vi "GageAverage.vi"() -> ()   [LabVIEW 2016]
uses:
  <vilib>/express/express analysis/Spectral/Block/exnSpectralBlock spectral measurements power poly.vi
  <vilib>/express/express analysis/Spectral/Block/exnSpectralBlock spectral measurements power WFM.vi
  <vilib>/Utility/file.llb/Write To Spreadsheet File (DBL).vi
  <vilib>/Analysis/2dsp.llb/1D Cross Correlation (DBL).vi
  <vilib>/express/express analysis/Spectral/XNode/ExpressSpectralMeasurementsBlockNode.xnode
  <vilib>/Analysis/NI_AALPro.lvlib
panel:
  out "100 세트 저장완료":bool
  in  "데이터 저장 시작":bool
  out "루프 사이의 time interval":dbl
  out "Ant 3":dbl(graph)
  out "ANt 2":dbl(graph)
  out "Ant 1":dbl(graph)
  in  "상호상관 샘플 갯수":dbl
  in  "상호상관\n채널 2":i32=1
  in  "상호상관 채널 1":i32=1
  out "웨이브폼 그래프 2":dbl[](graph)
  in  "표시 채널":i32=1
  out "웨이브폼 그래프":cluster{"f0":dbl, "df":dbl, "magnitude":dbl[]}(graph)
  in  "Trigger":T1={"Slope"=0, "Level"=0, "Source"=0, "External Range"=2000, "External Coupling"=0, "External"=FALSE, "Disable"=FALSE, "External Impedance"=1} {"External Impedance" items=["50 Ohm", "HiZ"]; "External Coupling" items=["DC", "AC"]; "External Range" min=2000 max=10000 step=8000; "Slope" items=["Rising", "Falling"]; "Level" min=-100 max=100; "Source" min=0 max=64 step=1}
  in  "Averages":u32=1 min=1 step=1
  in  "Averaging Method":bool
  in  "Channels":T2(array[cluster])=[{"Coupling"=0, "Differential Input"=FALSE, "Direct-to-ADC"=FALSE, "Range"=2000, "Impedance"=50, "Filter"=0}] {"Impedance" min=50 max=1000000 step=999950; "Coupling" items=["DC", "AC"]}
  in  "Acquisition":T3={"Sample Rate"=50000000.0, "Mode"=2, "Depth"=8192.0, "Segment Size"=8192.0, "Trigger Timeout"=1000000.0, "Trigger Holdoff"=0.0, "Trigger Delay"=0.0, "Clock mode"=enum."Internal"} {"Segment Size" min=256.0 step=128.0; "Trigger Holdoff" min=0.0 step=128.0; "Trigger Delay" min=0.0 step=128.0; "Depth" min=256.0 step=128.0; "Mode" items=["Single", "Dual", "Quad", "Octal"]}
  in  "Continuous":bool=TRUE
  out "Progress":string
  in  "stop":bool
  out "Waveform Graph":cluster{dbl, dbl, dbl[]}(graph)
  out "System Name":string
  out "Sample Bits":i32
  out "Trigger Count":i32
  out "Channel Count":i32
  out "Board Count":i32
  out "System Count":i32
  in  "Points":u32=4096
  in  "Start":i32
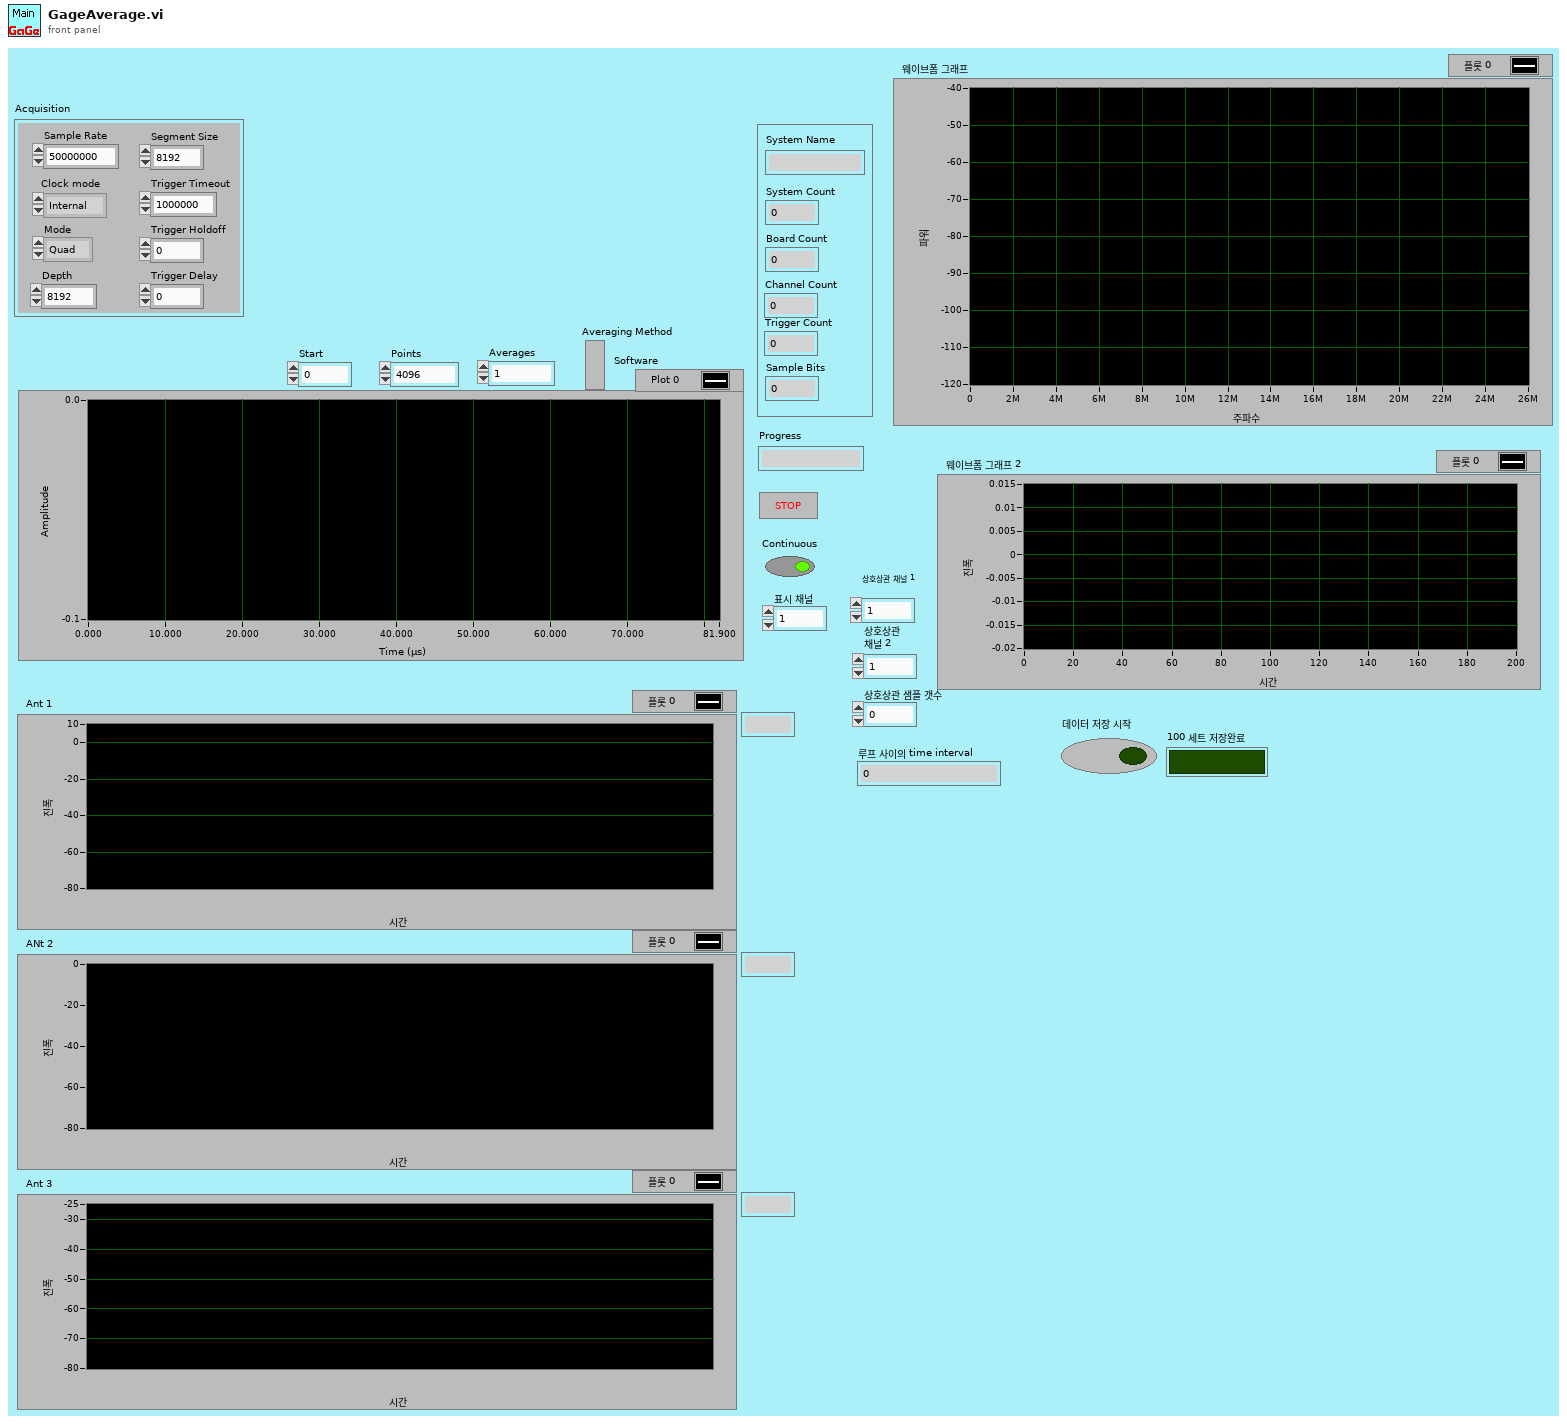
[diagram p1: front panel]
types:
  T1 = cluster{"Slope":u16, "Level":i32, "Source":i32, "External Range":u32, "External Coupling":u16, "External":bool, "Disable":bool, "External Impedance":u16}
  T2 = cluster{"Coupling":u16, "Differential Input":bool, "Direct-to-ADC":bool, "Range":u32, "Impedance":u32, "Filter":i32}[]
  T3 = cluster{"Sample Rate":dbl, "Mode":u16, "Depth":dbl, "Segment Size":dbl, "Trigger Timeout":dbl, "Trigger Holdoff":dbl, "Trigger Delay":dbl, "Clock mode":enum16{"Internal", "External", "Reference"}}
  T4 = cluster{"averaging mode":u16, "weighting mode":u16, "number of averages":u32}
  T5 = cluster{"dB On (F)":bool, "unwrap phase (F)":bool, "convert to degree (F)":bool}
  T6 = cluster{"Handle":u32, "Sample size":u32, "Resolution":i32, "Offset":i32, "Channels":u32, "Boards":u32}
  T7 = cluster{string, "Differential Input":bool, "Direct-to-ADC":bool, "Range":u32, "Impedance":u32, i32, "Filter":i32}
  T8 = cluster{"RingText.Text":string, "Level":i32, "Source":i32, "External Range":u32, "RingText.Text":string, "External":bool, "Disable":bool, "RingText.Text":string}
  T9 = cluster{"RingText.Text":string, "Level":i32, "Source":i32, "External Range":u32, "RingText.Text":string, "External":bool, "Disable":bool, "RingText.Text":string}[]
  T10 = cluster{"Handle":u32, "Sample Size":u32, "Resolution":i32, "Offset":i32, "Channels":u32, "Boards":u32}
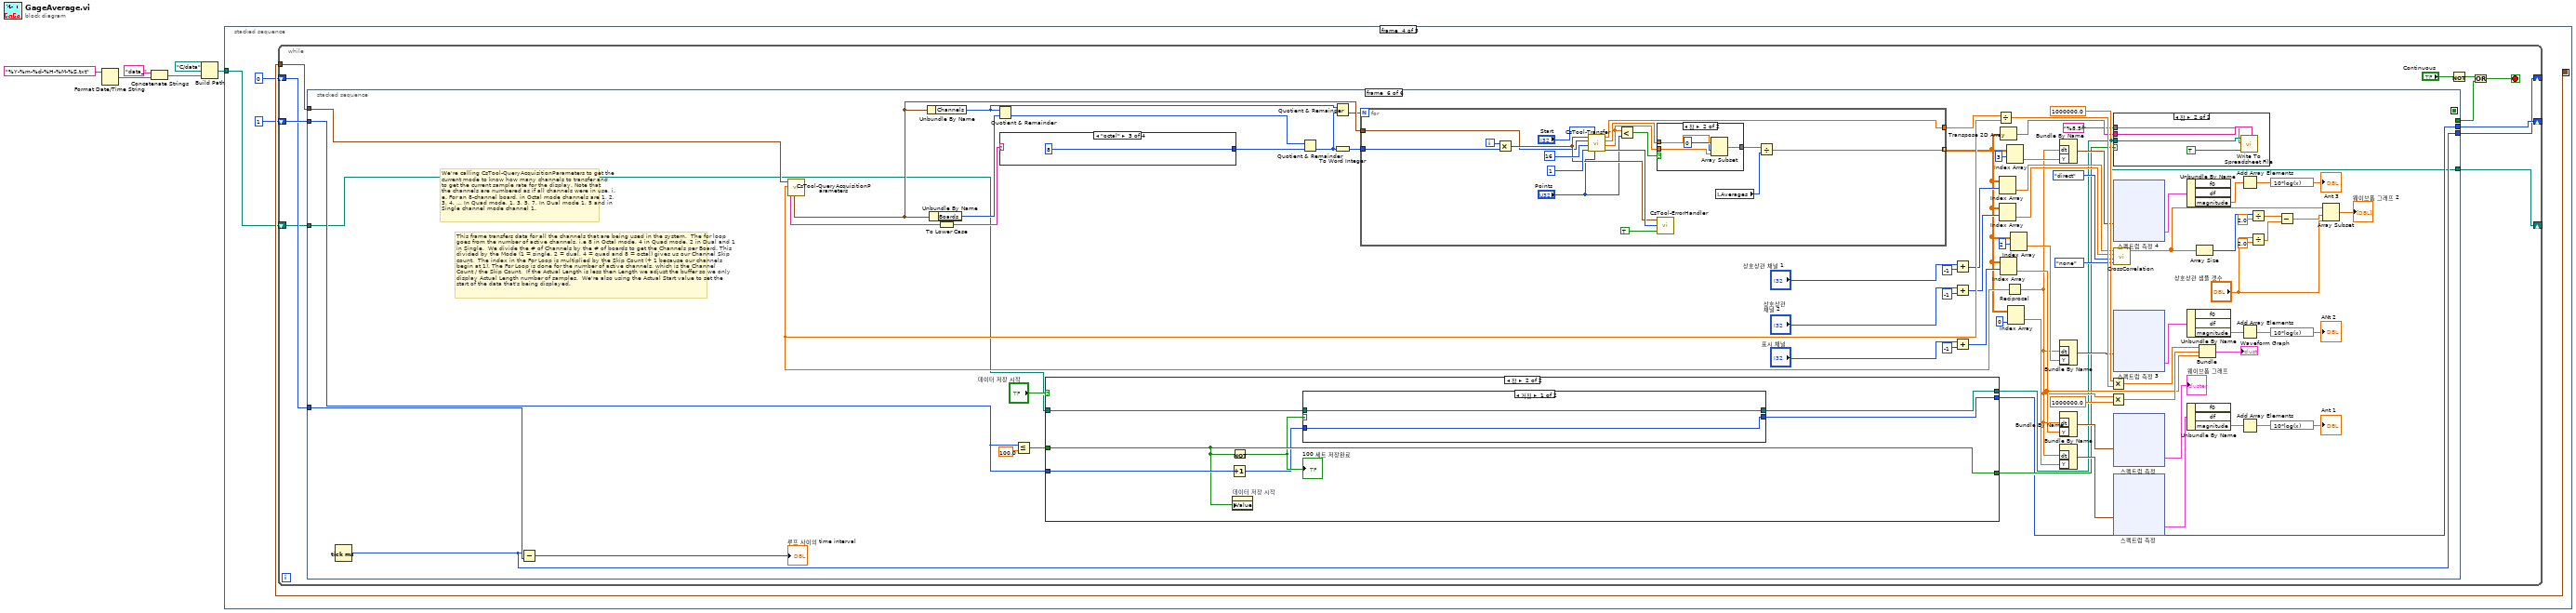
[diagram p0: block diagram]
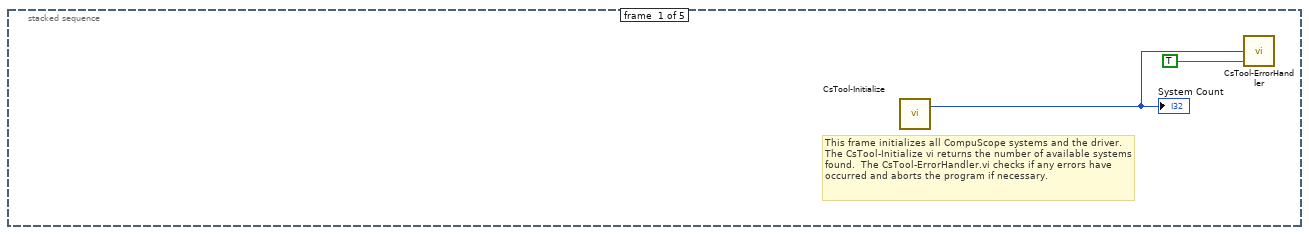
[diagram p2: hidden frame]
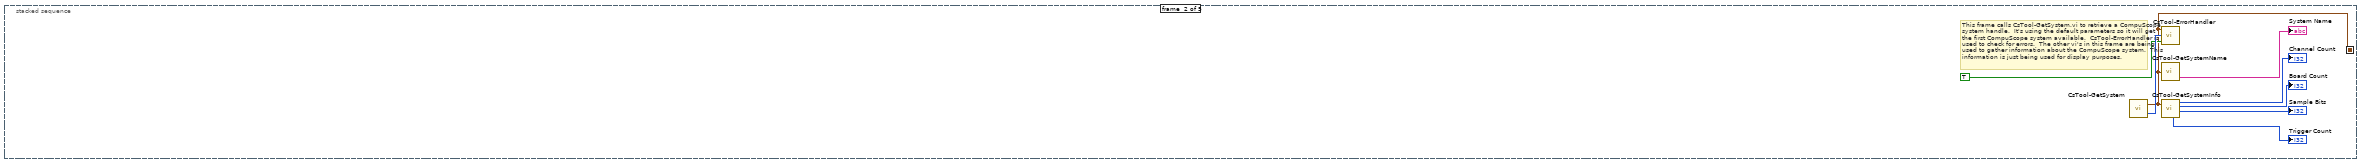
[diagram p3: hidden frame]
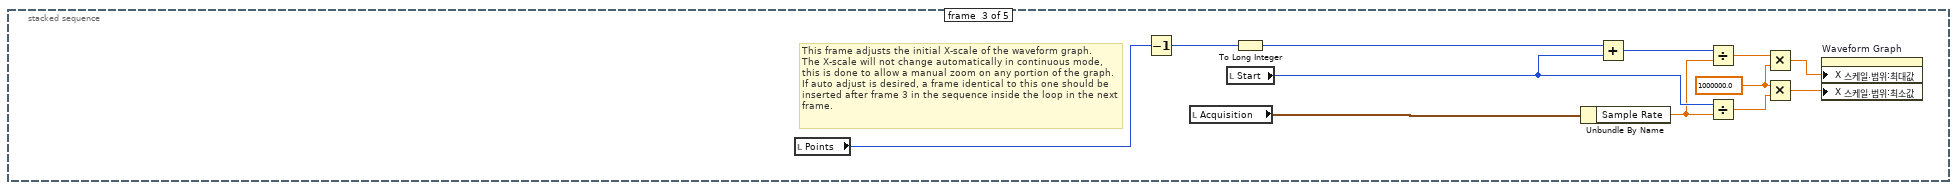
[diagram p4: hidden frame]
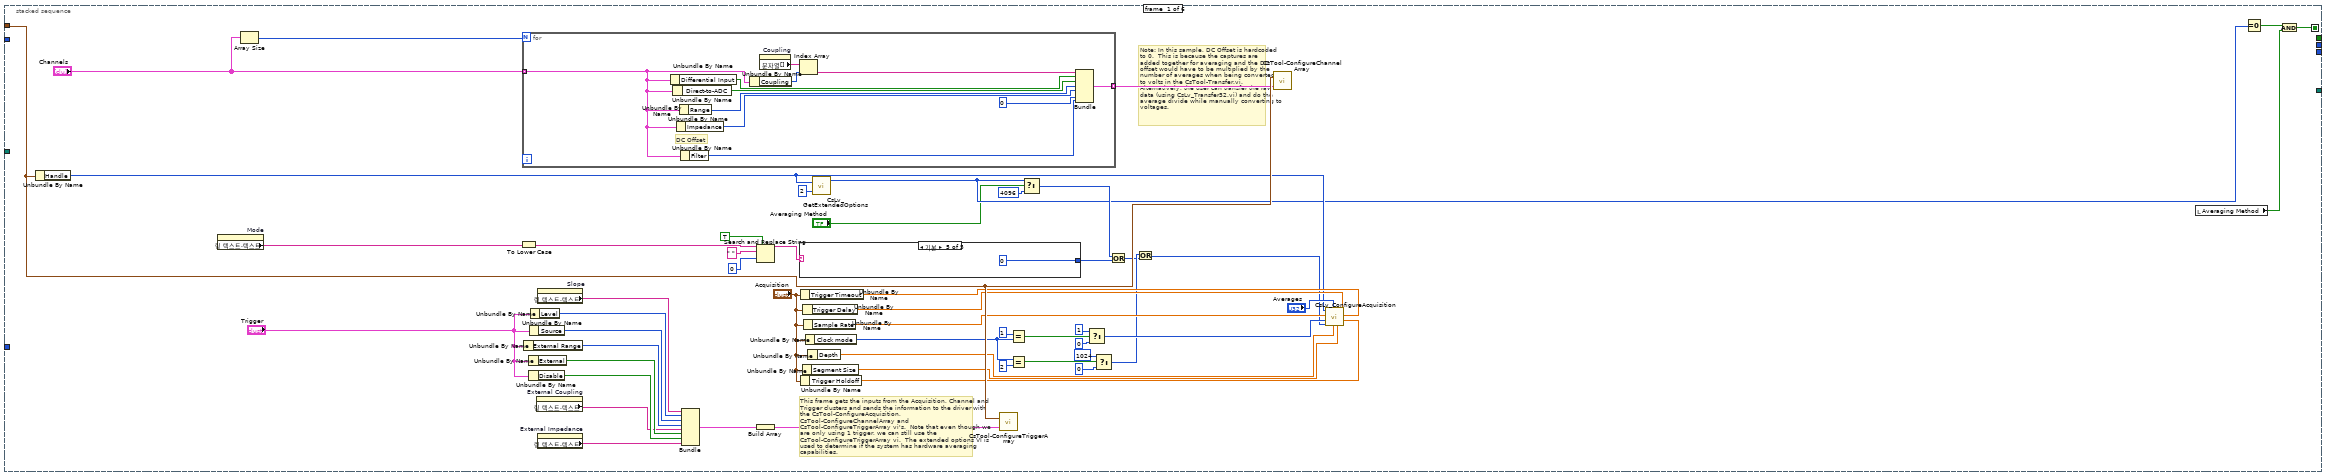
[diagram p5: hidden frame]
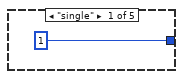
[diagram p6: hidden frame]
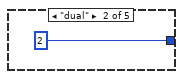
[diagram p7: hidden frame]
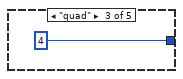
[diagram p8: hidden frame]
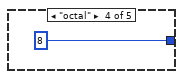
[diagram p9: hidden frame]
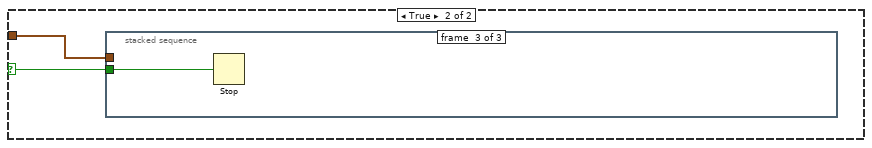
[diagram p11: hidden frame]
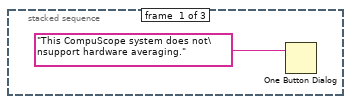
[diagram p12: hidden frame]
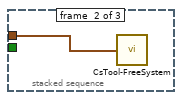
[diagram p13: hidden frame]
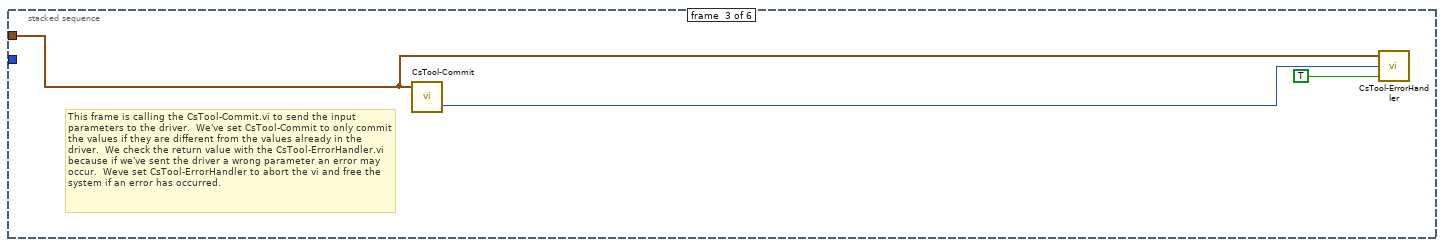
[diagram p14: hidden frame]
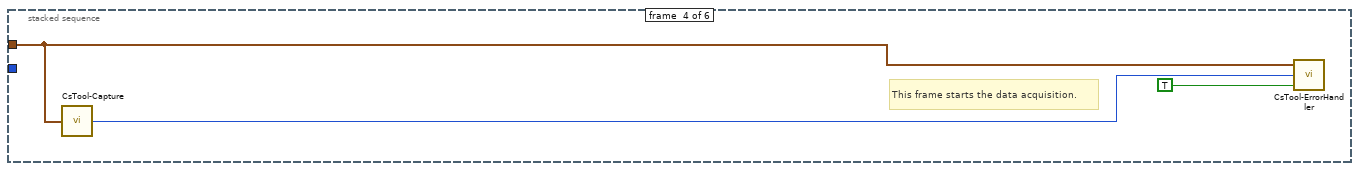
[diagram p15: hidden frame]
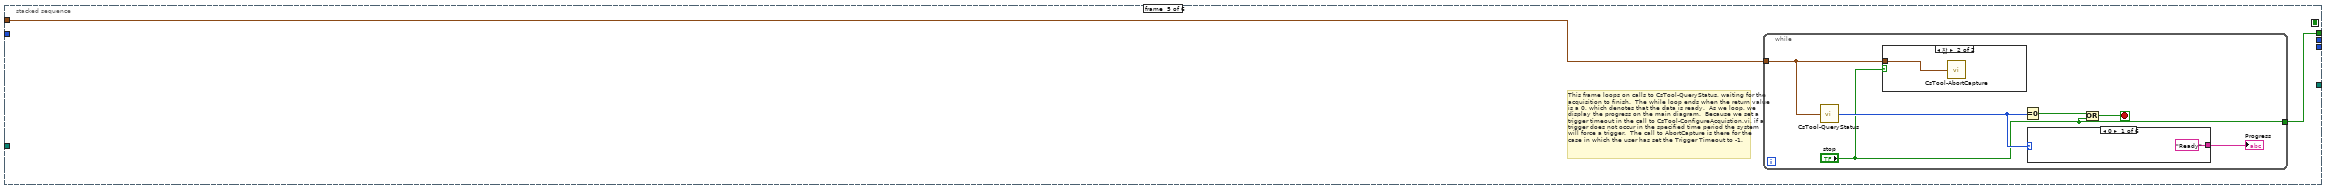
[diagram p16: hidden frame]
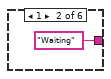
[diagram p18: hidden frame]
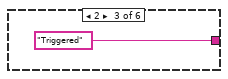
[diagram p19: hidden frame]
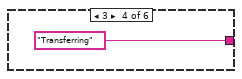
[diagram p20: hidden frame]
diagram:
  n1 = Format Date/Time String(time format string (%c)="%Y-%m-%d-%H-%M-%S.txt" ("시간 포맷 문자열 (%c)")) -> (date/time string=w2:string)  [unwired: 2 in]
  n2 = Concatenate Strings("data_", w2) -> (w1:string)
  n3 = Build Path(base path=path "C:/data", name or relative path=w1) -> (appended path=w4:path)
  n4 = stacked-sequence {
    seq-local: [_ w11 _ _ _] -> [_ _ _ w32 w305]
    tunnel: w4 -> [_ _ _ w29 _]
    frame #0 {
      # "This frame initializes all CompuScope systems and the driver.\nThe CsTool-Initialize vi returns the number of available systems found.  The CsTool-ErrorHandler.vi checks if any errors have occurred and aborts the program if necessary."
      n5 = call <userlib>:"CsTool-Initialize.vi"() -> ("Number Of Systems"=w8:i32)  [unwired: 1 out]
      "System Count" <- w8
      n6 = call <userlib>:"CsTool-ErrorHandler.vi"("StopOnError (true)"=TRUE, "Error Code"=w8) -> ()  [unwired: 1 in, 1 out]
    }
    frame #1 {
      # "This frame calls CsTool-GetSystem.vi to retrieve a CompuScope system handle.  It's using the default parameters so it will get the first CompuScope system available.  CsTool-ErrorHandler is used to check for errors.  The other vi's in this frame are being used to gather information about the CompuScope system.  This information is just being used for display purposes."
      n7 = call <userlib>:"CsTool-GetSystem.vi"() -> ("Error Code"=w13:i32, "Handle Cluster"=w11:T6)  [unwired: 4 in]
      n8 = call <userlib>:"CsTool-ErrorHandler.vi"("StopOnError (true)"=TRUE, "Error Code"=w13, "Handle Cluster"=w11) -> ()  [unwired: 1 out]
      n9 = call <userlib>:"CsTool-GetSystemName.vi"("Handle Cluster"=w11) -> ("System Name"=→"System Name":string)  [unwired: 1 out]
      n10 = call <userlib>:"CsTool-GetSystemInfo.vi"("Handle Cluster"=w11) -> ("Number Of Triggers"=→"Trigger Count":u32, "Number Of Channels"=→"Channel Count":u32, "Number Of Boards"=→"Board Count":u32, "Sample Bits"=→"Sample Bits":u32)  [unwired: 3 out]
    }
    frame #2 {
      w28 = 1000000.0
      # "This frame adjusts the initial X-scale of the waveform graph.\nThe X-scale will not change automatically in continuous mode, \nthis is done to allow a manual zoom on any portion of the graph.\nIf auto adjust is desired, a frame identical to this one should be\ninserted after frame 3 in the sequence inside the loop in the next frame."
      n11 = local read "Points"() -> (w23:u32)
      n12 = Decrement(x=w23) -> (x-1=w17:u32)
      n13 = local read "Acquisition"() -> (w21:T3)
      n14 = local read "Start"() -> (w24:i32)
      n15 = To Long Integer(number=w17) -> (32bit integer=w18:i32)
      n16 = Unbundle By Name(w21) -> ("Sample Rate"=w22:dbl)
      n17 = Add(x=w18, y=w24) -> (x+y=w20:i32)
      n18 = Divide(x=w20, y=w22) -> (x/y=w19:dbl)
      n19 = Divide(x=w24, y=w22) -> (x/y=w27:dbl)
      n20 = Multiply(x=w19, y=w28) -> (x*y=w25:dbl)
      n21 = Multiply(x=w28, y=w27) -> (x*y=w26:dbl)
      n22 = property on="Waveform Graph" class="WFGraph (엄격한)"("X 스케일.범위:최대값"=w25, "X 스케일.범위:최소값"=w26) -> ()  [unwired: 2 in, 2 out]
    }
    frame #3 {
      n23 = while {
        tunnel: w32 -> [w43]
        shift-right: [w37] -> _
        shift-left: 1 -> [w38]
        shift-right: [w35] -> _
        shift-left: 0 -> [w36]
        shift-right: [w34] -> _
        shift-left: w29 -> [w33]
        stop <- w40 stop-if-true
        n24 = stacked-sequence {
          seq-local: [w64 _ _ _ _ _] -> [_ w113 _ _ _ _]
          tunnel: w43 -> [w89 w112 w119 w122 w126 w219]
          tunnel: [_ _ _ _ w125 _] -> w39
          tunnel: w38 -> [_ _ _ _ _ w149]
          tunnel: [_ _ _ _ _ w150] -> w37
          tunnel: w36 -> [_ _ _ _ _ w156]
          tunnel: [_ _ _ _ _ w154] -> w35
          tunnel: [_ _ _ _ _ w144] -> w34
          tunnel: w33 -> [_ _ _ _ _ w143]
          frame #0 {
            # "Note: In this sample, DC Offset is hardcoded to 0.  This is because the captures are added together for averaging and the DC offset would have to be multiplied by the number of averages when being converted to volts in the CsTool-Transfer.vi. Alternatively, the user can transfer the raw data (using CsLv_Transfer32.vi) and do the average divide while manually converting to voltages."
            # "This frame gets the inputs from the Acquisition, Channel and Trigger clusters and sends the information to the driver with the CsTool-ConfigureAcquisition, CsTool-ConfigureChannelArray and CsTool-ConfigureTriggerArray vi's.  Note that even though we are only using 1 trigger, we can still use the CsTool-ConfigureTriggerArray vi.  The extended options VI is used to determine if the system has hardware averaging capabilities."
            n25 = Unbundle By Name(w89) -> ("Handle"=w68:u32)
            n26 = property on="Mode" class="Ring (엄격한)"() -> ("링 텍스트.텍스트"=w78:string)  [unwired: 2 in, 2 out]
            n27 = Array Size(array="Channels") -> (size(s)=w90:i32)
            n28 = To Lower Case(string=w78) -> (all lower case string=w84:string)
            n29 = for {
              N: w90 -> [_]
              tunnel: "Channels" -> [w103] mode=indexing
              tunnel: [w107] -> w48 mode=indexing
              # "DC Offset"
              n30 = Unbundle By Name(w103) -> ("Differential Input"=w111:bool)
              n31 = Unbundle By Name(w103) -> ("Direct-to-ADC"=w110:bool)
              n32 = Unbundle By Name(w103) -> ("Impedance"=w108:u32)
              n33 = Unbundle By Name(w103) -> ("Range"=w109:u32)
              n34 = Unbundle By Name(w103) -> ("Filter"=w102:i32)
              n35 = Unbundle By Name(w103) -> ("Coupling"=w105:u16)
              n36 = property on="Coupling" class="Ring (엄격한)"() -> ("문자열[]"=w106:string[])  [unwired: 2 in, 2 out]
              n37 = Index Array(array=w106, index=w105) -> (element=w104:string)
              n38 = Bundle(w104, "Differential Input"=w111, "Direct-to-ADC"=w110, "Range"=w109, "Impedance"=w108, 0, "Filter"=w102) -> (w107:T7)  [unwired: 1 in]
            }
            n39 = Unbundle By Name("Trigger") -> ("External Range"=w94:u32)
            n40 = Unbundle By Name("Trigger") -> ("External"=w50:bool)
            n41 = Unbundle By Name("Trigger") -> ("Disable"=w49:bool)
            n42 = Unbundle By Name("Trigger") -> ("Source"=w51:i32)
            n43 = Unbundle By Name("Trigger") -> ("Level"=w95:i32)
            n44 = property on="External Coupling" class="Ring (엄격한)"() -> ("링 텍스트.텍스트"=w45:string)  [unwired: 2 in, 2 out]
            n45 = property on="Slope" class="Ring (엄격한)"() -> ("링 텍스트.텍스트"=w46:string)  [unwired: 2 in, 2 out]
            n46 = property on="External Impedance" class="Ring (엄격한)"() -> ("링 텍스트.텍스트"=w44:string)  [unwired: 2 in, 2 out]
            n47 = Bundle("RingText.Text"=w46, "Level"=w95, "Source"=w51, "External Range"=w94, "RingText.Text"=w45, "External"=w50, "Disable"=w49, "RingText.Text"=w44) -> (w93:T8)  [unwired: 1 in]
            n48 = Search and Replace String(replace all?=TRUE, input string=w84, search string=" ", offset=0) -> (result string=w81:string)  [unwired: 4 in, 3 out]
            n49 = Build Array(w93) -> (w92:T9)
            n50 = case shown="기본" w81 {
              tunnel: [1 2 4 8 0] -> w69
              frame "single" {
              }
              frame "dual" {
              }
              frame "quad" {
              }
              frame "octal" {
              }
              frame Default {
              }
            }
            n51 = Unbundle By Name("Acquisition") -> ("Trigger Timeout"=w75:dbl)
            n52 = Unbundle By Name("Acquisition") -> ("Trigger Holdoff"=w74:dbl)
            n53 = Unbundle By Name("Acquisition") -> ("Segment Size"=w77:dbl)
            n54 = Unbundle By Name("Acquisition") -> ("Trigger Delay"=w76:dbl)
            n55 = Unbundle By Name("Acquisition") -> ("Sample Rate"=w88:dbl)
            n56 = Unbundle By Name("Acquisition") -> ("Clock mode"=w59:enum16{"Internal", "External", "Reference"})
            n57 = Unbundle By Name("Acquisition") -> ("Depth"=w80:dbl)
            n58 = call <userlib>:"CsLv_GetExtendedOptions.vi"("Handle"=w68, "Option"=2) -> ("User Mode"=w66:u32)  [unwired: 2 out]
            n59 = call <userlib>:"CsTool-ConfigureTriggerArray.vi"("Triggers"=w92, "Handle Cluster"=w89) -> ()  [unwired: 1 out]
            n60 = Equal?(x=1, y=w59) -> (x = y?=w60:bool)
            n61 = Equal?(x=w59, y=2) -> (x = y?=w57:bool)
            n62 = Select(t=w66, s="Averaging Method", f=4096) -> (s? t:f=w70:u32)
            n63 = Select(t=u32 1, s=w60, f=u32 0) -> (s? t:f=w85:u32)
            n64 = Select(t=1024, s=w57, f=0) -> (s? t:f=w56:i32)
            n65 = Or(x=w70, y=w69) -> (x .or. y?=w54:u32)
            n66 = Or(x=w56, y=w54) -> (x .or. y?=w55:u32)
            n67 = call <userlib>:"CsTool-ConfigureChannelArray.vi"("Channels"=w48, "Handle Cluster"=w89) -> ()  [unwired: 1 out]
            n68 = call <userlib>:"CsLv_ConfigureAcquisition.vi"("Trigger Holdoff (0)"=w74, "Trigger Timeout (10000000)"=w75, "Trigger Delay (0)"=w76, "Segment Size (8192)"=w77, "Depth (8192)"=w80, "Segment Count (1)"="Averages", "Mode (2)"=w55, "External Clock (0)"=w85, "Sample Rate (100000000)"=w88, "Handle"=w68) -> ()  [unwired: 1 in, 1 out]
            n69 = local read "Averaging Method"() -> (w53:bool)
            n70 = Equal To 0?(x=w66) -> (x = 0?=w65:bool)
            n71 = And(x=w65, y=w53) -> (x .and. y?=w64:bool)
          }
          frame #1 {
            # "If, in the previous frame, the CsLv_GetExtendedOptions vi returned a 0, this means that hardware averaging is not available for this system. So if hardware averaging was chosend and the system does not support it, we will report the error, free the CompuScope system and stop the application."
            n72 = case shown="거짓" w113 {
              selector: w113 -> [_ w114]
              tunnel: w112 -> [_ w115]
              frame False {
              }
              frame True {
                n73 = stacked-sequence {
                  tunnel: w115 -> [_ w117 _]
                  tunnel: w114 -> [_ _ w118]
                  frame #0 {
                    n74 = One Button Dialog(message="This CompuScope system does not\nsupport hardware averaging.") -> ()  [unwired: 1 in, 1 out]
                  }
                  frame #1 {
                    n75 = call <userlib>:"CsTool-FreeSystem.vi"("Handle Cluster"=w117) -> ()  [unwired: 1 out]
                  }
                  frame #2 {
                    n76 = Stop(stop? (T)=w118) -> ()
                  }
                }
              }
            }
          }
          frame #2 {
            # "This frame is calling the CsTool-Commit.vi to send the input parameters to the driver.  We've set CsTool-Commit to only commit the values if they are different from the values already in the driver.  We check the return value with the CsTool-ErrorHandler.vi because if we've sent the driver a wrong parameter an error may occur.  Weve set CsTool-ErrorHandler to abort the vi and free the system if an error has occurred."
            n77 = call <userlib>:"CsTool-Commit.vi"("Handle Cluster"=w119) -> ("Error Code"=w121:i32)  [unwired: 2 in, 1 out]
            n78 = call <userlib>:"CsTool-ErrorHandler.vi"("StopOnError (true)"=TRUE, "Error Code"=w121, "Handle Cluster"=w119) -> ()  [unwired: 1 out]
          }
          frame #3 {
            # "This frame starts the data acquisition."
            n79 = call <userlib>:"CsTool-Capture.vi"("Handle Cluster"=w122) -> ("Error Code"=w124:i32)
            n80 = call <userlib>:"CsTool-ErrorHandler.vi"("StopOnError (true)"=TRUE, "Error Code"=w124, "Handle Cluster"=w122) -> ()  [unwired: 1 out]
          }
          frame #4 {
            # "This frame loops on calls to CsTool-QueryStatus, waiting for the acquisition to finish.  The while loop ends when the return value is a 0, which denotes that the data is ready.  As we loop, we display the progress on the main diagram.  Because we set a trigger timeout in the call to CsTool-ConfigureAcquistion.vi, if a trigger does not occur in the specified time period the system will force a trigger.  The call to AbortCapture is there for the case in which the user has set the Trigger Timeout to -1."
            n81 = while {
              tunnel: w126 -> [w127]
              tunnel: ["stop"] -> w125
              stop <- w129 stop-if-true
              n82 = call <userlib>:"CsTool-QueryStatus.vi"("Handle Cluster"=w127) -> ("Status"=w132:i32)
              n83 = case shown="참" "stop" {
                tunnel: w127 -> [_ w133]
                frame False {
                }
                frame True {
                  n84 = call <userlib>:"CsTool-AbortCapture.vi"("Handle Cluster"=w133) -> ()  [unwired: 1 out]
                }
              }
              n85 = Equal To 0?(x=w132) -> (x = 0?=w130:bool)
              n86 = case shown="0" w132 {
                tunnel: ["Ready" "Waiting" "Triggered" "Transferring" "Calibrating" " "] -> w131
                frame 0 {
                }
                frame 1 {
                }
                frame 2 {
                }
                frame 3 {
                }
                frame 4 {
                }
                frame 5, Default {
                }
              }
              "Progress" <- w131
              n87 = Or(x=w130, y="stop") -> (x .or. y?=w129:bool)
            }
          }
          frame #5 {
            # "We're calling CsTool-QueryAcquisitionParameters to get the current mode to know how many channels to transfer and to get the current sample rate for the display. Note that the channels are numbered as if all channels were in use, i.e. For an 8-channel board, in Octal mode channels are 1, 2, 3, 4, ... In Quad mode, 1, 3, 5, 7. In Dual mode 1, 5 and in Single channel mode channel 1."
            # "This frame transfers data for all the channels that are being used in the system.  The for loop goes from the number of active channels, i.e 8 in Octal mode, 4 in Quad mode, 2 in Dual and 1 in Single.  We divide the # of Channels by the # of boards to get the Channels per Board. This divided by the Mode (1 = single, 2 = dual, 4 = quad and 8 = octal) gives us our Channel Skip count.  The index in the For Loop is multiplied by the Skip Count (+ 1 because our channels begin at 1). The For Loop is done for the number of active channels, which is the Channel Count / the Skip Count.  If the Actual Length is less then Length we adjust the buffer so we only display Actual Length number of samples.  We're also using the Actual Start value to set the start of the data that's being displayed."
            n88 = Tick Count (ms)() -> (millisecond timer value=w154:u32)
            n89 = Subtract(x=w154, y=w156) -> (x-y=→"루프 사이의 time interval":u32)
            n90 = call <userlib>:"CsTool-QueryAcquisitionParameters.vi"("Handle Cluster"=w219) -> ("Output Handle Cluster"=w218:T10, "Mode"=w210:string, "Sample Rate"=w202:dbl)  [unwired: 8 out]
            n91 = Unbundle By Name(w218) -> ("Channels"=w205:u32)
            n92 = Unbundle By Name(w218) -> ("Boards"=w208:u32)
            n93 = To Lower Case(string=w210) -> (all lower case string=w209:string)
            n94 = Quotient & Remainder(x=w205, y=w208) -> (floor(x/y)=w207:u32)  [unwired: 1 out]
            n95 = case shown="\"octal\"" w209 {
              tunnel: [2 4 8 1] -> w206
              frame "dual", Default {
              }
              frame "quad" {
              }
              frame "octal" {
              }
              frame "single" {
              }
            }
            n96 = Less Or Equal?(x=w149, y=100.0) -> (x <= y?=w152:bool)
            n97 = case shown="참" "데이터 저장 시작" {
              tunnel: [FALSE w228] -> w151
              tunnel: w152 -> [_ w228]
              tunnel: [w222 w225] -> w150
              tunnel: w149 -> [w222 w229]
              tunnel: w143 -> [w220 w224]
              tunnel: [w220 w223] -> w144
              frame False {
              }
              frame True {
                n98 = Increment(x=w229) -> (x+1=w226:i32)
                n99 = Not(x=w228) -> (.not. x?=w227:bool)
                "100 세트 저장완료" <- w227
                n100 = property on="데이터 저장 시작" class="Bool (엄격한)"("Value"=w228) -> ()  [unwired: 2 in, 2 out]
                n101 = case shown="거짓" w227 {
                  tunnel: [w231 1] -> w225
                  tunnel: w226 -> [w231 _]
                  tunnel: w224 -> [w230 _]
                  tunnel: [w230 w232] -> w223
                  frame False {
                  }
                  frame True {
                    n102 = Format Date/Time String(time format string (%c)="%Y-%m-%d-%H-%M-%S.txt" ("시간 포맷 문자열 (%c)")) -> (date/time string=w234:string)  [unwired: 2 in]
                    n103 = Concatenate Strings("data_", w234) -> (w233:string)
                    n104 = Build Path(base path=path "C:/data", name or relative path=w233) -> (appended path=w232:path)
                  }
                }
              }
            }
            n105 = Quotient & Remainder(x=w207, y=w206) -> (floor(x/y)=w204:u32)  [unwired: 1 out]
            n106 = Quotient & Remainder(x=w205, y=w204) -> (floor(x/y)=w203:u32)  [unwired: 1 out]
            n107 = To Word Integer(number=w204) -> (16bit integer=w217:i16)
            n108 = for {
              N: w203 -> [_]
              tunnel: [w296] -> w216
              tunnel: w218 -> [w288]
              tunnel: [w284] -> w166 mode=indexing
              tunnel: w217 -> [w289]
              i -> [w298]
              n109 = Multiply(x=w298, y=w289) -> (x*y=w287:i32)
              n110 = call <userlib>:"CsTool-Transfer.vi"("Length (4096)"="Points", "Start (0)"="Start", "Segment (1)"=1, "Mode (0)"=16, "Channel (0)"=w287, "Handle Cluster"=w288) -> ("Error Code"=w292:i32, "Actual Length"=w295:dbl, "Data in Volts"=w285:dbl[], "Actual Start"=w296:dbl)
              n111 = Less?(x=w295, y="Points") -> (x < y?=w299:bool)
              n112 = case shown="참" w299 {
                tunnel: w285 -> [w300 w304]
                tunnel: w295 -> [_ w302]
                tunnel: [w300 w301] -> w286
                frame False {
                }
                frame True {
                  n113 = Array Subset(array=w304, index=0, length=w302) -> (w301:dbl[])
                }
              }
              n114 = call <userlib>:"CsTool-ErrorHandler.vi"("StopOnError (true)"=TRUE, "Error Code"=w292, "Handle Cluster"=w288) -> ()  [unwired: 1 out]
              n115 = local read "Averages"() -> (w290:u32)
              n116 = Divide(x=w286, y=w290) -> (x/y=w284:dbl[])
            }
            n117 = Add(x="상호상관 채널 1", y=-1) -> (x+y=w187:i32)
            n118 = Add(x="상호상관\n채널 2", y=-1) -> (x+y=w188:i32)
            n119 = Add(x="표시 채널", y=-1) -> (x+y=w196:i32)
            n120 = Divide(x=w216, y=w202) -> (x/y=w215:dbl)
            n121 = Index Array(array=w166, index (row)=w187) -> (element=w181:dbl[])  [unwired: 1 in]
            n122 = Index Array(array=w166, index (row)=w188) -> (element=w180:dbl[])  [unwired: 1 in]
            n123 = Transpose 2D Array(2D array=w166) -> (transposed array=w158:dbl[][])
            n124 = Index Array(array=w166, index (row)=w196) -> (element=w195:dbl[])  [unwired: 1 in]
            n125 = Reciprocal(x=w202) -> (1/x=w165:dbl)
            n126 = Index Array(array=w166, index (row)=3 ("인덱스 (행)")) -> (element=w169:dbl[])  [unwired: 1 in]
            n127 = Index Array(array=w166, index (col)=0 ("비활성화된 인덱스 (열)")) -> (element=w177:dbl[])  [unwired: 1 in]
            n128 = Index Array(array=w166, index (row)=2 ("인덱스 (행)")) -> (element=w173:dbl[])  [unwired: 1 in]
            n129 = Bundle By Name("dt"=w165, "Y"=w169) -> (w170:waveform(dbl))  [unwired: 1 in]
            n130 = Bundle By Name("dt"=w165, "Y"=w173) -> (w174:waveform(dbl))  [unwired: 1 in]
            n131 = Bundle By Name("dt"=w165, "Y"=w195) -> (w199:waveform(dbl))  [unwired: 1 in]
            n132 = Bundle By Name("dt"=w165, "Y"=w177) -> (w178:waveform(dbl))  [unwired: 1 in]
            n133 = Multiply(x=1000000.0, y=w215) -> (x*y=w213:dbl)
            n134 = Multiply(x=w165, y=1000000.0) -> (x*y=w211:dbl)
            n135 = case shown="참" w151 {
              tunnel: w144 -> [_ w242]
              tunnel: "%8.5f" ("format (%.3f)") -> [_ w240]
              tunnel: w158 -> [_ w239]
              frame False {
              }
              frame True {
                n136 = call-poly <vilib>:"Write To Spreadsheet File.vi"("format (%.3f)"=w240, "append to file? (new file:F)"=TRUE, "2D data"=w239, "file path (dialog if empty)"=w242) -> ()  [unwired: 4 in, 1 out]
              }
            }
            n137 = xnode "스펙트럼 측정 4"("신호"=w170) -> ("파워 스펙트럼"=w168:cluster{"f0":dbl, "df":dbl, "magnitude":dbl[]})  [unwired: 1 in, 1 out]
            n138 = call-poly <vilib>:"CrossCorrelation.vi"("normalization"=enum32{"none", "unbiased", "biased"}."none", "algorithm"=enum32{"direct", "frequency domain"}."direct", "Y"=w180, "X"=w181) -> ("Rxy"=w148:dbl[])  [unwired: 6 in, 1 out]
            n139 = xnode "스펙트럼 측정 3"("신호"=w174) -> ("파워 스펙트럼"=w172:cluster{"f0":dbl, "df":dbl, "magnitude":dbl[]})  [unwired: 1 in, 1 out]
            n140 = xnode "스펙트럼 측정"("신호"=w199) -> ("파워 스펙트럼"=→"웨이브폼 그래프":cluster{"f0":dbl, "df":dbl, "magnitude":dbl[]})  [unwired: 1 in, 1 out]
            n141 = xnode "스펙트럼 측정"("신호"=w178) -> ("파워 스펙트럼"=w176:cluster{"f0":dbl, "df":dbl, "magnitude":dbl[]})  [unwired: 1 in, 1 out]
            n142 = Unbundle By Name(w168) -> ("magnitude"=w167:dbl[])  [unwired: 2 out]
            n143 = Unbundle By Name(w172) -> ("magnitude"=w171:dbl[])  [unwired: 2 out]
            n144 = Unbundle By Name(w176) -> ("magnitude"=w175:dbl[])  [unwired: 2 out]
            n145 = Array Size(array=w148) -> (size(s)=w147:i32)
            n146 = Bundle(w213, w211, w195) -> (→"Waveform Graph":cluster{dbl, dbl, dbl[]})  [unwired: 1 in]
            n147 = Add Array Elements(numeric array=w167) -> (sum=w161:dbl)
            n148 = Add Array Elements(numeric array=w171) -> (sum=w160:dbl)
            n149 = Add Array Elements(numeric array=w175) -> (sum=w159:dbl)
            n150 = Divide(x=w147, y=2.0) -> (x/y=w145:dbl)
            n151 = Divide(x="상호상관 샘플 갯수", y=2.0) -> (x/y=w185:dbl)
            n152 = expression code="10*log(x)"(w161) -> (→"Ant 3":dbl)
            n153 = expression code="10*log(x)"(w160) -> (→"ANt 2":dbl)
            n154 = expression code="10*log(x)"(w159) -> (→"Ant 1":dbl)
            n155 = Subtract(x=w145, y=w185) -> (x-y=w186:dbl)
            n156 = Array Subset(array=w148, index=w186, length="상호상관 샘플 갯수") -> (→"웨이브폼 그래프 2":dbl[])
          }
        }
        n157 = Not(x="Continuous") -> (.not. x?=w42:bool)
        n158 = Or(x=w42, y=w39) -> (x .or. y?=w40:bool)
      }
    }
    frame #4 {
      # "This frame frees the handle associated with the CompuScope system we've been using.  This allows the system to be used by another application."
      n159 = call <userlib>:"CsTool-FreeSystem.vi"("Handle Cluster"=w305) -> ()  [unwired: 1 out]
    }
  }
